vi "MessageBase.getFieldSpecIndexByName.vi"(8 "error in (no error)":errorcluster, 10 "Field.Name":string="Length", 11 "MessageBase in":refnum<class "MessageBase.lvclass">) -> (0 "error out":errorcluster, 2 "Index":i32, 3 "MessageBase out":refnum<class "MessageBase.lvclass">)   [LabVIEW 2020, in "MessageBase.lvclass"]
uses:
  MessageBase.lvclass
  MessageBase.lvclass/MessageBase.ctl
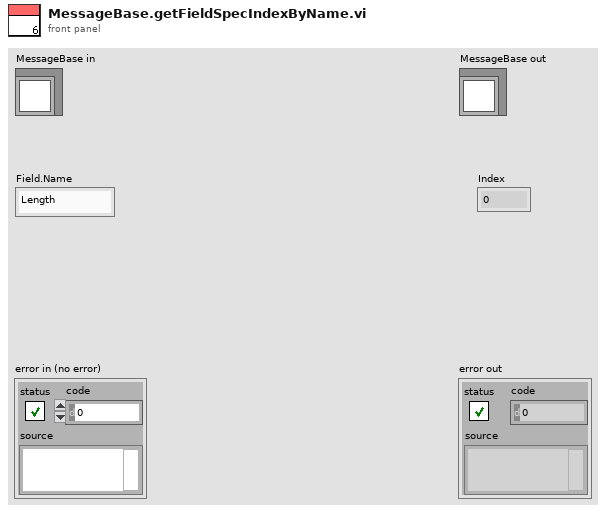
[diagram p1: front panel]
types:
  T1 = typedef "FieldSpec.ctl" = cluster{"Name":string, "Offset":i32, "Length":i32, "FieldType":enum16{"Alphanumeric", "Binary", "BinaryLongPrice", "BinaryShortPrice", "BitField", "PrintableAscii", "Value"}, "FieldValue":variant}
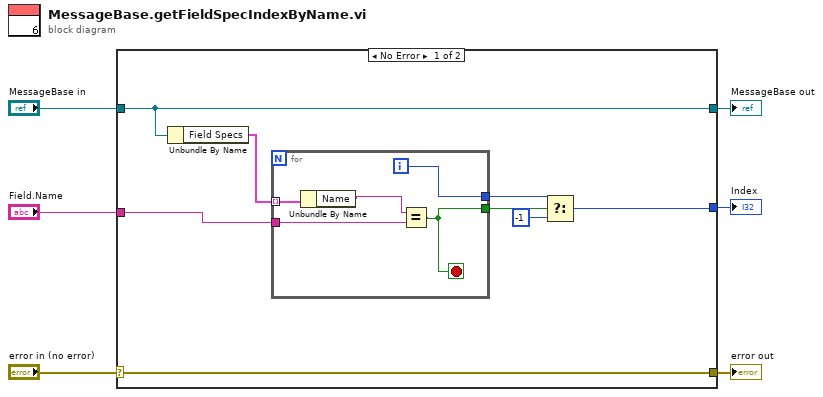
[diagram p0: block diagram]
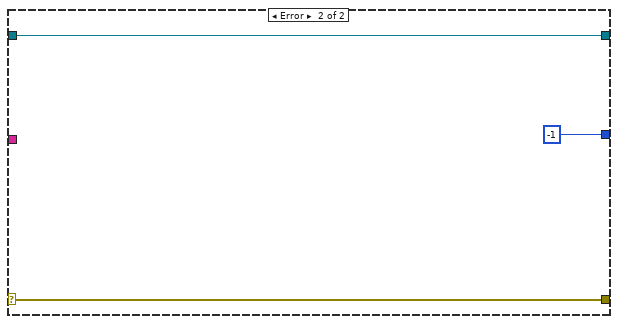
[diagram p2: hidden frame]
diagram:
  n1 = case shown="No Error" "error in (no error)" {
    selector: "error in (no error)" -> [w14 w22]
    tunnel: [w14 w22] -> w5
    tunnel: [w9 w21] -> w3
    tunnel: "MessageBase in" -> [w9 w21]
    tunnel: "Field.Name" -> [w8 _]
    tunnel: [w7 -1 ("f")] -> w1
    frame No Error {
      n2 = Unbundle By Name(w9) -> ("Field Specs"=w13:T1[])
      n3 = for {
        tunnel: w13 -> [w19] mode=indexing
        tunnel: [w17] -> w11
        tunnel: w8 -> [w16]
        tunnel: [w15] -> w12
        i -> [w17]
        stop <- w15 stop-if-true
        n4 = Unbundle By Name(w19) -> ("Name"=w18:string)
        n5 = Equal?(x=w18, y=w16) -> (x = y?=w15:bool)
      }
      n6 = Select(t=w11, s=w12, f=-1) -> (s? t:f=w7:i32)
    }
    frame Error {
    }
  }
  "error out" <- w5
  "MessageBase out" <- w3
  "Index" <- w1
